vi "Write Array.vi"(8 "error in (no error)":errorcluster, 10 "Array":u16[](array[ring]) items=["dev1", "5051"], 11 "Test Properties in":refnum<class "Test Properties.lvclass">) -> (0 "error out":errorcluster, 3 "Test Properties out":refnum<class "Test Properties.lvclass">)   [LabVIEW 2015, in "Test Properties.lvclass"]
uses:
  Test Properties.lvclass
  Test Properties.lvclass/Test Properties.ctl
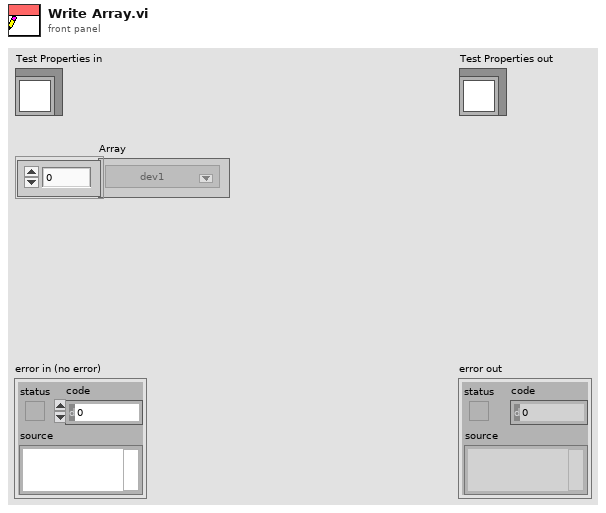
[diagram p1: front panel]
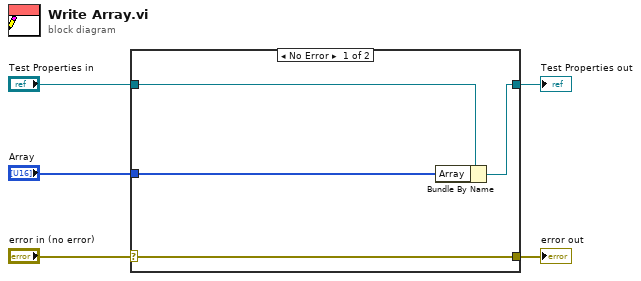
[diagram p0: block diagram]
diagram:
  n1 = case shown="No Error" "error in (no error)" {
    selector: "error in (no error)" -> [w9 w10]
    tunnel: [w9 w10] -> w4
    tunnel: [w7 w11] -> w2
    tunnel: "Test Properties in" -> [w8 w11]
    tunnel: "Array" -> [w6 _]
    frame No Error {
      n2 = Bundle By Name(cluster=w8, "Array"=w6) -> (w7:refnum<class "Test Properties.lvclass">)
    }
    frame Error {
    }
  }
  "error out" <- w4
  "Test Properties out" <- w2
